vi "WPI_DriverStationStart VI Asynchronous.vi"(11 "VI":refnum<vi>) -> (0 "error out":errorcluster, 3 "VI out":refnum<vi>)   [LabVIEW 2017]
doc: "This software is licensed. Open the labview\\readme\\WPI Robotics Library Open Source License.txt file for more information."
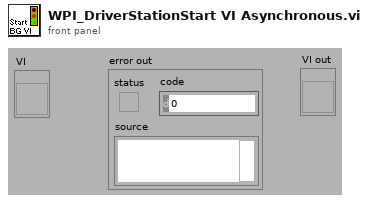
[diagram p1: front panel]
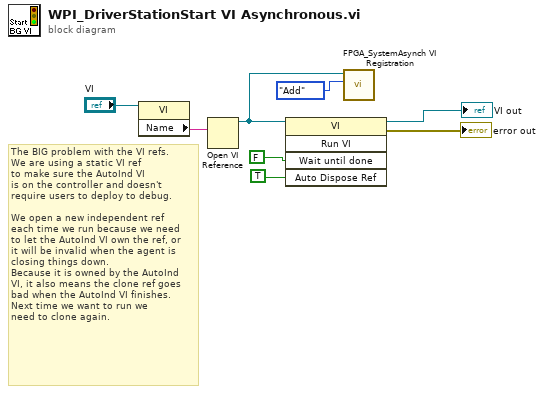
[diagram p0: block diagram]
diagram:
  # "The BIG problem with the VI refs.\nWe are using a static VI ref\nto make sure the AutoInd VI\nis on the controller and doesn't\nrequire users to deploy to debug.\n\nWe open a new independent ref\neach time we run because we need\nto let the AutoInd VI own the ref, or\nit will be invalid when the agent is\nclosing things down.\nBecause it is owned by the AutoInd\nVI, it also means the clone ref goes\nbad when the AutoInd VI finishes.\nNext time we want to run we\nneed to clone again."
  n1 = property class="VI"(reference="VI") -> ("Name"=w6:string)  [unwired: 1 in, 2 out]
  n2 = Open VI Reference(vi path=w6) -> (vi reference=w1:refnum<vi>)  [unwired: 2 in, 4 out]
  n3 = invoke class="VI" method="Run VI"(reference=w1, "Wait until done"=FALSE ("Wait Until Done"), "Auto Dispose Ref"=TRUE ("Wait Until Done")) -> (reference out=→"VI out":refnum<vi>, error out=→"error out":errorcluster)  [unwired: 2 in, 3 out]
  n4 = call <vilib>:"FPGA_SystemAsynch VI Registration.vi"("Operation"=enum16{"Get", "Add", "Remove"}."Add", "VI Refnum"=w1) -> ()  [unwired: 10 out]
